vi "main_example.vi"() -> ()   [LabVIEW 2010]
panel:
  in  "stop\nlistening loop":bool
  out "Distances\nBlue":dbl[](array[numeric])
  out "Distances\nRed":dbl[](array[numeric])
  out "Wheel turns\nRed":dbl
  out "Line sensors\nRed":dbl[](array[numeric])
  out "Wheel turns\nBlue":dbl
  out "Line sensors\nBlue":dbl[](array[numeric])
  in  "Steering value\nRed":u8
  in  "Motor value\nRed":u8=100
  in  "Steering value\nBlue":u8
  in  "Motor value\nBlue":u8=100
  in  "stop\ncontrol loop":bool
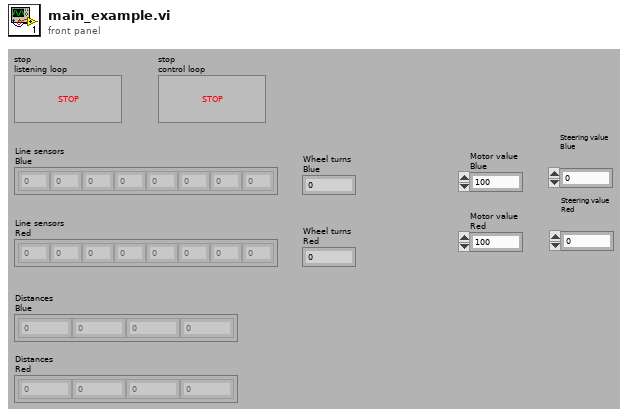
[diagram p1: front panel]
types:
  T1 = cluster{"Connected to\nsensors":bool, "connection ID\nsensors":refnum<k5>, "Connected to\nactuators":bool, "connection ID\nactuators":refnum<k5>}
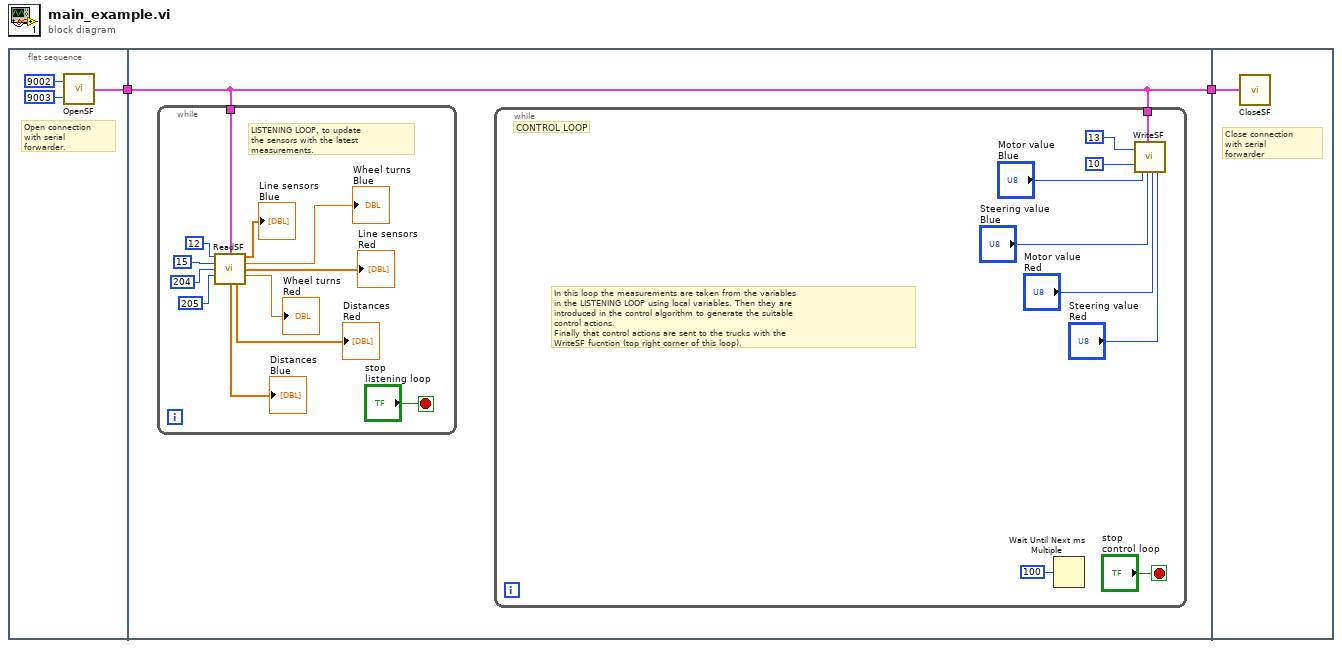
[diagram p0: block diagram]
diagram:
  n1 = flat-sequence {
    tunnel: [w3] -> w1
    tunnel: [w6] -> w2
    tunnel: w1 -> [w6]
    tunnel: w2 -> [w28]
    frame #0 {
      # "Open connection\nwith serial\nforwarder."
      n2 = call "OpenSF.vi"("Port number\nactuators"=u16 9003 ("Port number\nactuators"), "Port number\nsensors"=u16 9002 ("Port number\nsensors")) -> ("connection IDs"=w3:T1)
    }
    frame #1 {
      n3 = while {
        tunnel: w6 -> [w16]
        stop <- "stop\nlistening loop" stop-if-true
        # "LISTENING LOOP, to update\nthe sensors with the latest\nmeasurements."
        n4 = call "ReadSF.vi"("ID_sensor0\nBlue"=u16 12 ("ID_sensor0\nBlue"), "connection IDs"=w16, "ID_sensor0\nRed"=u16 15 ("ID_sensor0\nRed"), "ID_sensor1\nBlue"=u16 204 ("ID_sensor1\nBlue"), "ID_sensor1\nRed"=u16 205 ("ID_sensor1\nRed")) -> ("Line sensors\nBlue"=→"Line sensors\nBlue":dbl[], "Wheel turns\nBlue"=→"Wheel turns\nBlue":dbl, "Line sensors\nRed"=→"Line sensors\nRed":dbl[], "Wheel turns\nRed"=→"Wheel turns\nRed":dbl, "Distances\nBlue"=→"Distances\nBlue":dbl[], "Distances\nRed"=→"Distances\nRed":dbl[])  [unwired: 5 in]
      }
      n5 = while {
        tunnel: w6 -> [w20]
        stop <- "stop\ncontrol loop" stop-if-true
        # "In this loop the measurements are taken from the variables\nin the LISTENING LOOP using local variables. Then they are\nintroduced in the control algorithm to generate the suitable\ncontrol actions.\nFinally that control actions are sent to the trucks with the\nWriteSF fucntion (top right corner of this loop)."
        # "CONTROL LOOP"
        n6 = Wait Until Next ms Multiple(millisecond multiple=u32 100) -> ()  [unwired: 1 out]
        n7 = call "WriteSF.vi"("Actuator ID\nBlue"=u16 13 ("Actuator ID\nBlue"), "Actuator ID\nRed"=u16 10 ("Actuator ID\nRed"), "Motor value\nBlue"="Motor value\nBlue", "connection IDs"=w20, "Steering value\nBlue"="Steering value\nBlue", "Motor value\nRed"="Motor value\nRed", "Steering value\nRed"="Steering value\nRed") -> ()  [unwired: 13 in]
      }
    }
    frame #2 {
      # "Close connection\nwith serial \nforwarder"
      n8 = call "CloseSF.vi"("connection IDs"=w28) -> ()
    }
  }
